vi "Test MultiVal.vi"() -> ()   [LabVIEW 2012]
uses:
  Multivalue Buffer.xctl
panel:
  out "Numeric":i32
  in  "Stop":bool
  out "Multivalue Buffer":cluster{"Time":timestamp, "Val":dbl[]}(xcontrol)
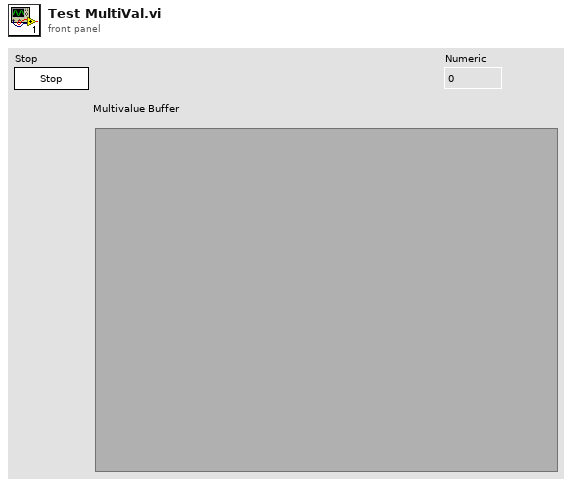
[diagram p1: front panel]
types:
  T1 = cluster{"seconds since 1Jan1904":timestamp, dbl[]}
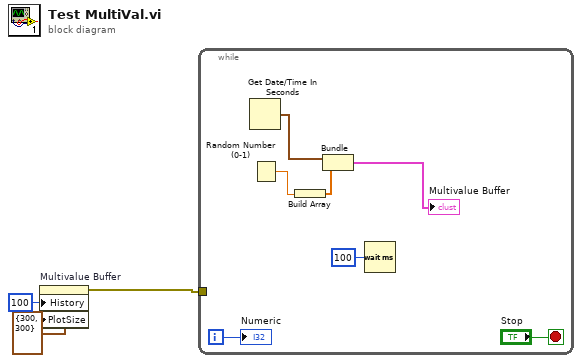
[diagram p0: block diagram]
diagram:
  n1 = property on="Multivalue Buffer" class="Multivalue Buffer (strict)"("History"=100, "PlotSize"=cluster{"Height":i32, "Width":i32} {"Height"=300, "Width"=300}) -> (error out=w2:errorcluster)  [unwired: 2 in, 1 out]
  n2 = while {
    tunnel: w2 -> [_]
    i -> [w4]
    stop <- "Stop" stop-if-true
    n3 = Get Date/Time In Seconds() -> (seconds since 1Jan1904=w10:timestamp)
    n4 = Random Number (0-1)() -> (number: 0 to 1=w9:dbl)
    n5 = Build Array(w9) -> (w8:dbl[])
    n6 = Bundle("seconds since 1Jan1904"=w10, w8) -> (→"Multivalue Buffer":T1)  [unwired: 1 in]
    n7 = Wait (ms)(milliseconds to wait=u32 100) -> ()  [unwired: 1 out]
    "Numeric" <- w4
  }
